vi "separate 3 section of QPD and position.vi"(6 "QPD signal (V)":dbl[](array[numeric]), 7 "X=T; Y=F":bool, 8 "stage position (um)":dbl[](array[numeric])) -> (0 "2nd section of QPD (V)":dbl[](array[numeric]), 1 "1st section of QPD (V)":dbl[](array[numeric]), 2 "3rd section of QPD (V)":dbl[](array[numeric]), 3 "3rd section of position (um)":dbl[](array[numeric]), 4 "1st section of position (um)":dbl[](array[numeric]), 5 "2nd section of position (um)":dbl[](array[numeric]))   [LabVIEW 2014]
panel:
  out "max value":dbl
  out "max index(es)":i32
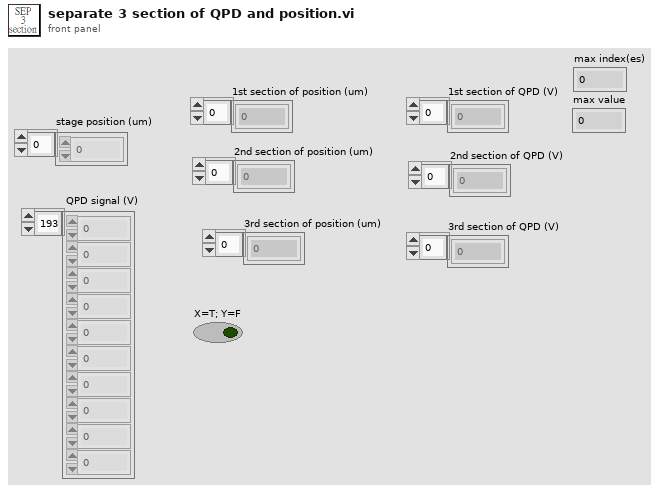
[diagram p1: front panel]
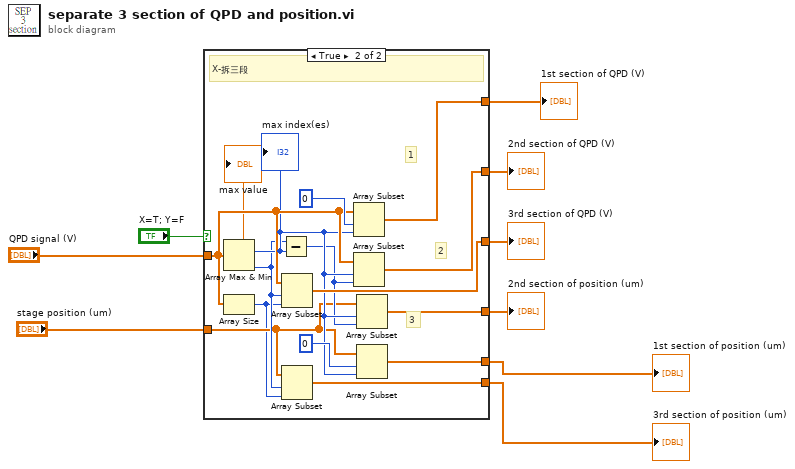
[diagram p0: block diagram]
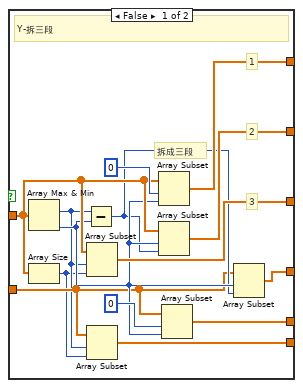
[diagram p2: hidden frame]
diagram:
  n1 = case shown="True" "X=T; Y=F" {
    tunnel: "QPD signal (V)" -> [w19 w34]
    tunnel: [w22 w37] -> w5
    tunnel: [w21 w36] -> w2
    tunnel: [w20 w35] -> w1
    tunnel: "stage position (um)" -> [w13 w27]
    tunnel: [w17 w32] -> w6
    tunnel: [w14 w29] -> w4
    tunnel: [w11 w25] -> w3
    frame False {
      # "拆成三段"
      # "3"
      # "2"
      # "1"
      # "Y-拆三段"
      n2 = Array Max & Min(array=w19) -> (max index (indices)=w12:i32, min index (indices)=w16:i32)  [unwired: 2 out]
      n3 = Array Size(array=w19) -> (size(s)=w10:i32)
      n4 = Subtract(x=w12, y=w16) -> (x-y=w15:i32)
      n5 = Array Subset(array=w19, index=w12, length=w10) -> (w20:dbl[])
      n6 = Array Subset(array=w13, index=w12, length=w10) -> (w11:dbl[])
      n7 = Array Subset(array=w19, index=0, length=w16) -> (w22:dbl[])
      n8 = Array Subset(array=w19, index=w16, length=w15) -> (w21:dbl[])
      n9 = Array Subset(array=w13, index=0, length=w16) -> (w17:dbl[])
      n10 = Array Subset(array=w13, index=w16, length=w15) -> (w14:dbl[])
    }
    frame True {
      # "3"
      # "2"
      # "1"
      # "X-拆三段"
      n11 = Array Max & Min(array=w34) -> (max value=→"max value":dbl, max index (indices)=w31:i32, min index (indices)=w28:i32)  [unwired: 1 out]
      "max index(es)" <- w31
      n12 = Array Size(array=w34) -> (size(s)=w26:i32)
      n13 = Subtract(x=w28, y=w31) -> (x-y=w30:i32)
      n14 = Array Subset(array=w34, index=w28, length=w26) -> (w35:dbl[])
      n15 = Array Subset(array=w27, index=w28, length=w26) -> (w25:dbl[])
      n16 = Array Subset(array=w34, index=0, length=w31) -> (w37:dbl[])
      n17 = Array Subset(array=w34, index=w31, length=w30) -> (w36:dbl[])
      n18 = Array Subset(array=w27, index=w31, length=w30) -> (w29:dbl[])
      n19 = Array Subset(array=w27, index=0, length=w31) -> (w32:dbl[])
    }
  }
  "1st section of position (um)" <- w6
  "1st section of QPD (V)" <- w5
  "2nd section of position (um)" <- w4
  "3rd section of position (um)" <- w3
  "2nd section of QPD (V)" <- w2
  "3rd section of QPD (V)" <- w1
